vi "eFGV - Modbus Reply Alarm.vi"(6 "State - eFGV":T3=enum."Close", 8 "error in (no error)":errorcluster, 10 "Event Message":T1) -> (0 "error out":errorcluster, 2 "Event - Modbus Event Msg":refnum<user-event>)   [LabVIEW 2019]
uses:
  Control/State - eFGV.ctl
  Control/Data Struct - Device Event Msg.ctl
  Control/Device Name.ctl
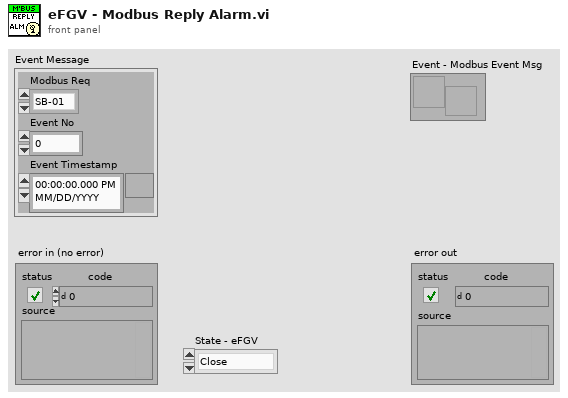
[diagram p1: front panel]
types:
  T1 = typedef "Data Struct - Device Event Msg.ctl" = cluster{"Modbus Req":T2, "Event No":u32, "Event Timestamp":timestamp}
  T2 = typedef "Device Name.ctl" = enum16{"SB-01", "SB-02", "SB-03", "SB-04", "STP-01", "STP-02", "STP-03", "STP-04", "BANK-01", "BANK-02", "BANK-03", "BANK-04", "SI-M-01", "SI-M-02", "SI-M-03", "SI-M-04", "PM-01", "PM-02", "PM-03", "PM-04"}
  T3 = typedef "State - eFGV.ctl" = enum16{"Init", "Read", "Write", "Close"}
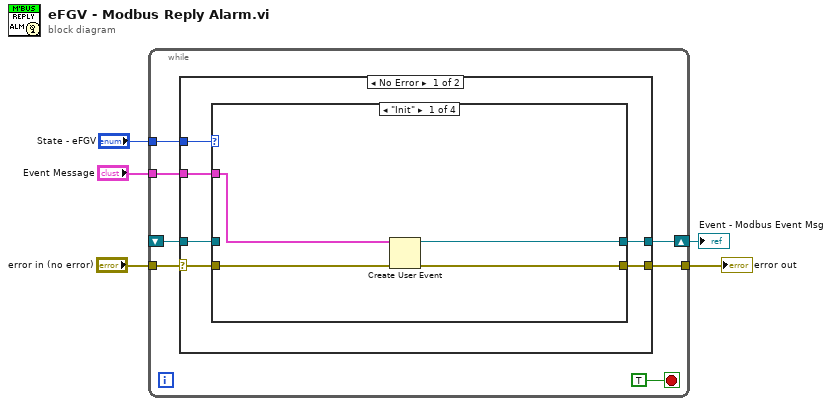
[diagram p0: block diagram]
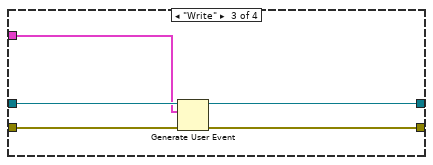
[diagram p3: hidden frame]
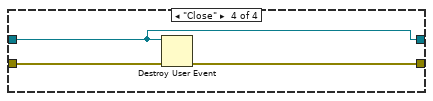
[diagram p4: hidden frame]
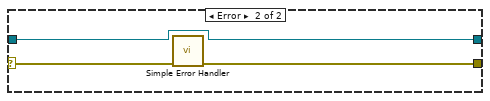
[diagram p5: hidden frame]
diagram:
  n1 = while {
    tunnel: "State - eFGV" -> [w11]
    tunnel: "error in (no error)" -> [w10]
    tunnel: [w9] -> w3
    tunnel: "Event Message" -> [w8]
    shift-right: [w7] -> w1
    shift-left: _ -> [w6]
    stop <- TRUE stop-if-true
    n2 = case shown="No Error" w10 {
      selector: w10 -> [w17 w35]
      tunnel: w11 -> [w18 _]
      tunnel: [w16 w34] -> w9
      tunnel: w8 -> [w15 _]
      tunnel: [w14 w33] -> w7
      tunnel: w6 -> [w13 w33]
      frame No Error {
        n3 = case shown="\"Init\"" w18 {
          tunnel: w17 -> [w22 w24 w29 w32]
          tunnel: [w21 w24 w28 w31] -> w16
          tunnel: w15 -> [w20 _ w26 _]
          tunnel: [w19 w23 w25 w30] -> w14
          tunnel: w13 -> [_ w23 w27 w30]
          frame "Init" {
            n4 = Create User Event(user event datatype=w20, error in=w22) -> (user event=w19:refnum<user-event>, error out=w21:errorcluster)
          }
          frame "Read", Default {
          }
          frame "Write" {
            n5 = Generate User Event(user event=w27, event data cluster=w26, error in=w29) -> (user event out=w25:refnum<user-event>, error out=w28:errorcluster)  [unwired: 1 in]
          }
          frame "Close" {
            n6 = Destroy User Event(user event=w30, error in=w32) -> (error out=w31:errorcluster)
          }
        }
      }
      frame Error {
        n7 = call <vilib>:"Simple Error Handler.vi"("error in (no error)"=w35) -> ("error out"=w34:errorcluster)  [unwired: 4 in, 4 out]
      }
    }
  }
  "error out" <- w3
  "Event - Modbus Event Msg" <- w1
